vi "Get Handler by Name.vi"(8 "error in":errorcluster, 10 "Name":string, 11 "Logger in":refnum<class "Logger.lvclass">) -> (0 "error out":errorcluster, 2 "Handler out":refnum<class "Handler.lvclass">, 3 "Logger out":refnum<class "Logger.lvclass">)   [LabVIEW 2020, in "hse-logger.lvlib" / "Logger.lvclass"]
doc: "Returns the handler with the specified name.\nIf name was not found, returns a basis handler without functionality and raise an error \"510802 - Handler name not found\".\n\n____\nHAMPEL SOFTWARE ENGINEERING v2.0.6 (2021-04-15 11:38)"
uses:
  Logger.lvclass
  Handler/Handler.lvclass
  Logger.lvclass/Logger.ctl
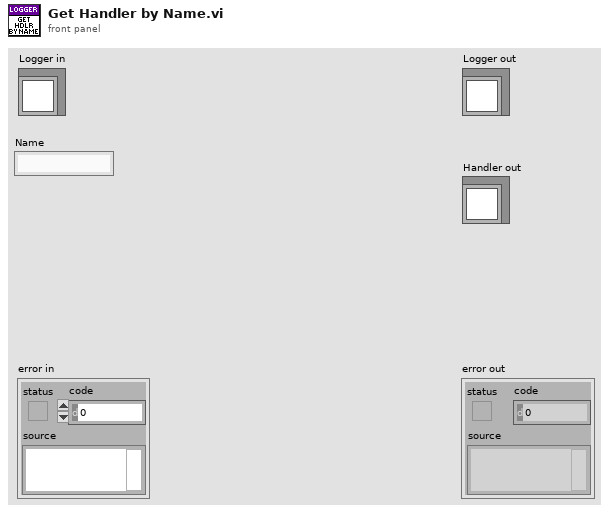
[diagram p1: front panel]
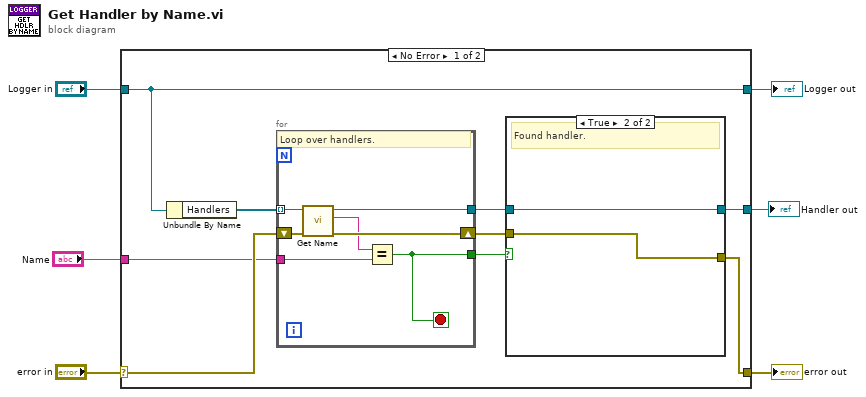
[diagram p0: block diagram]
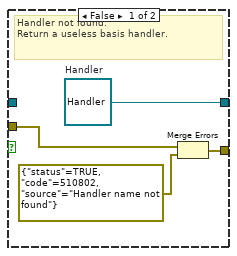
[diagram p2: hidden frame]
diagram:
  n1 = case shown="No Error" "error in" {
    selector: "error in" -> [w13 w30]
    tunnel: [w7 w30] -> w5
    tunnel: [w15 w29] -> w3
    tunnel: "Logger in" -> [w15 w29]
    tunnel: "Name" -> [w12 _]
    tunnel: [w8 _] -> w1
    frame No Error {
      n2 = Unbundle By Name(w15) -> ("Handlers"=w14:refnum<class "Handler.lvclass">[])
      n3 = for {
        tunnel: w14 -> [w27] mode=indexing
        tunnel: w12 -> [w25]
        tunnel: [w23] -> w11
        shift-right: [w28] -> w10
        shift-left: w13 -> [w26]
        tunnel: [w22] -> w9
        stop <- w23 stop-if-true
        # "Loop over handlers."
        n4 = call-dynamic "Get Name.vi"("error in"=w26, "Handler in"=w27) -> ("error out"=w28:errorcluster, "Name"=w24:string, "Handler out"=w22:refnum<class "Handler.lvclass">)  [unwired: 7 in]
        n5 = Equal?(x=w24, y=w25) -> (x = y?=w23:bool)
      }
      n6 = case shown="True" w11 {
        tunnel: w10 -> [w18 w20]
        tunnel: w9 -> [_ w21]
        tunnel: [w19 w21] -> w8
        tunnel: [w16 w20] -> w7
        frame False {
          w19 = refnum<class "Handler.lvclass"> refnum  # Handler
          # "Handler not found.\nReturn a useless basis handler."
          n7 = Merge Errors(w18, errorcluster {"status"=TRUE, "code"=510802, "source"="Handler name not found"} ("error out")) -> (w16:errorcluster)
        }
        frame True {
          # "Found handler."
        }
      }
    }
    frame Error {
    }
  }
  "error out" <- w5
  "Logger out" <- w3
  "Handler out" <- w1
